vi "Create File.vi"(8 "error in (no error)":errorcluster, 10 "File Name Prefix":string) -> (0 "error out":errorcluster, 3 "refnum out":refnum<file>)   [LabVIEW 2015]
uses:
  <vilib>/Utility/sysdir.llb/System Directory Type.ctl
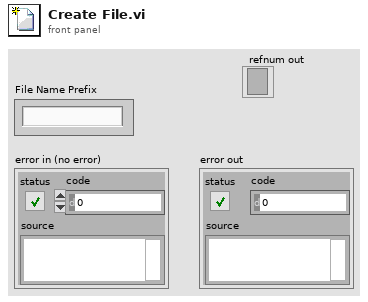
[diagram p1: front panel]
types:
  T1 = typedef "System Directory Type.ctl" = i32
  T2 = enum16{"open", "replace", "create", "open or create", "replace or create", "replace or create with confirmation"}
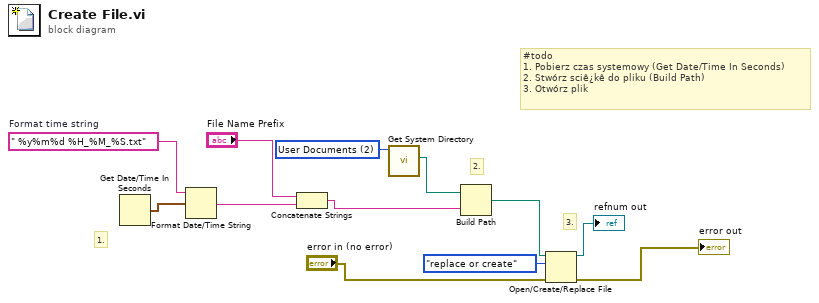
[diagram p0: block diagram]
diagram:
  w1 = T1 2 items=["User Home"=0, "User Desktop"=1, "User Documents"=2, "User Application Data"=3, "User Preferences"=4, "User Temporary"=5, "Public Documents"=6, "Public Application Data"=7, "Public Preferences"=8, "Public Cache"=13, "System Core Libraries"=9, "System Installed Libraries"=10, "Application Files"=11, "Boot Volume Root"=12] ("system directory type")
  w11 = " %y%m%d %H_%M_%S.txt"  # Format time string
  # "3."
  # "2."
  # "1."
  # "#todo\n1. Pobierz czas systemowy (Get Date/Time In Seconds)\n2. Stwórz sciê¿kê do pliku (Build Path)\n3. Otwórz plik"
  n1 = Get Date/Time In Seconds() -> (seconds since 1Jan1904=w5:timestamp)
  n2 = Format Date/Time String(time format string (%c)=w11, seconds (now)=w5) -> (date/time string=w12:string)  [unwired: 1 in]
  n3 = Concatenate Strings("File Name Prefix", w12) -> (w9:string)
  n4 = call <vilib>:"Get System Directory.vi"("system directory type"=w1) -> ("system directory"=w2:path)  [unwired: 10 in]
  n5 = Build Path(base path=w2, name or relative path=w9) -> (appended path=w8:path)
  n6 = Open/Create/Replace File(file path (use dialog)=w8, error in="error in (no error)", operation (0:open)=T2."replace or create") -> (refnum out=→"refnum out":refnum<file>, error out=→"error out":errorcluster)  [unwired: 3 in, 1 out]
